vi "parser.vi"(0 "in string":string, 3 "variables":dbl[](array[numeric])=[0.0, 0.0, 0.0], 4 "leaves":string[](array[string])=["Cube", "Pyramid", "Sphere"]) -> (5 "leaves_projection_array":cluster{"matrix":dbl[][], "leave":string}[](array[cluster])=[{"matrix"=[[100.0, -1.3951473992034527e-14, -1.3951473992034527e-14, 0.0], [1.3951473992034527e-14, 100.0, -1.3951473992034527e-14, 0.0], [1.3951473992034527e-14, 1.3951473992034527e-14, 100.0, 0.0], [0.0, 0.0, 0.0, 1.0]], "leave"="Pyramid"}, {"matrix"=[[10.0, -6.975736996017264e-16, -6.975736996017264e-16, 146.93877551020412], [6.975736996017264e-16, 10.0, -6.975736996017264e-16, 10.00000000000001], [6.975736996017264e-16, 6.975736996017264e-16, 10.0, 10.00000000000001], [0.0, 0.0, 0.0, 1.0]], "leave"="Cube"}, {"matrix"=[[10.0, -6.975736996017264e-16, -6.975736996017264e-16, 9.999999999999996], [6.975736996017264e-16, 10.0, -6.975736996017264e-16, 50.0], [6.975736996017264e-16, 6.975736996017264e-16, 10.0, 10.000000000000004], [0.0, 0.0, 0.0, 1.0]], "leave"="Cube"}] {"matrix" format="%#.6f"})   [LabVIEW 2011]
uses:
  <vilib>/Analysis/baseanly.llb/Real A x B.vi
  <vilib>/Analysis/NI_AALBase.lvlib
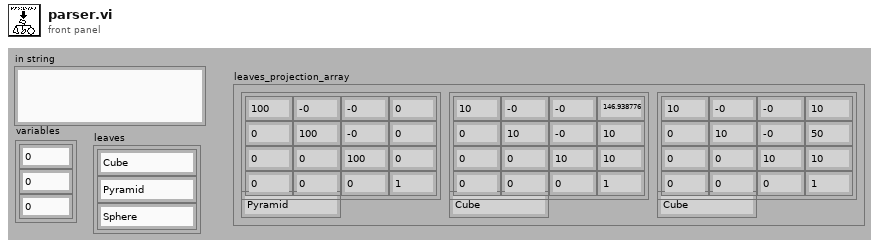
[diagram p1: front panel]
types:
  T1 = typedef "NI_Matrix.lvlib/RealMatrix.ctl" = dbl[][]
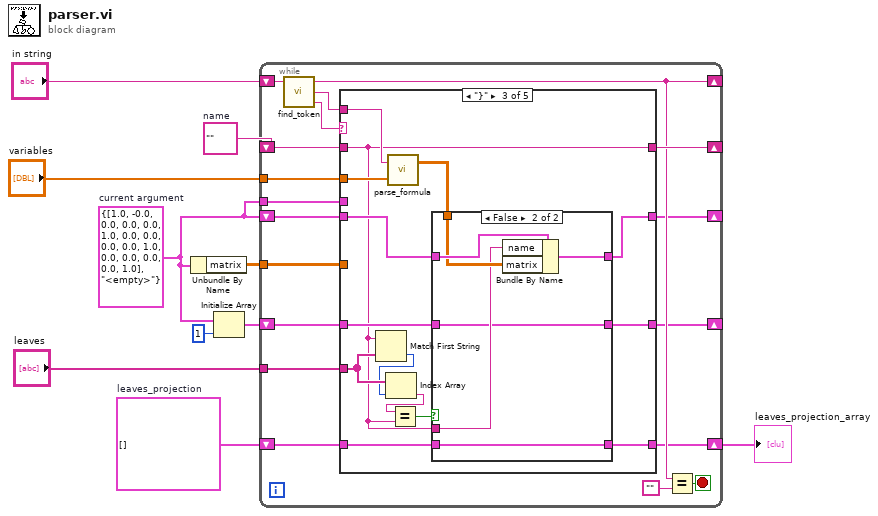
[diagram p0: block diagram]
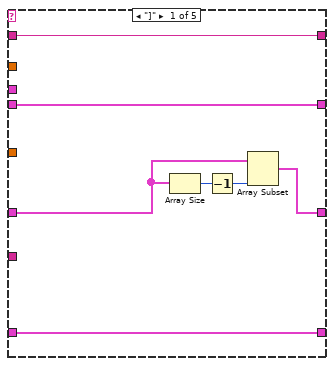
[diagram p2: hidden frame]
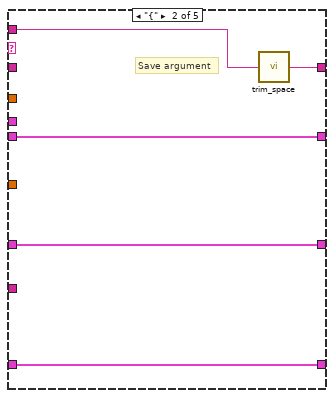
[diagram p3: hidden frame]
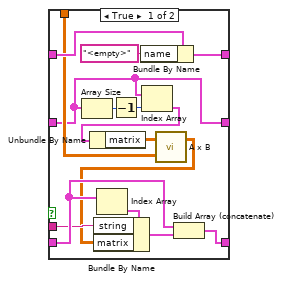
[diagram p4: hidden frame]
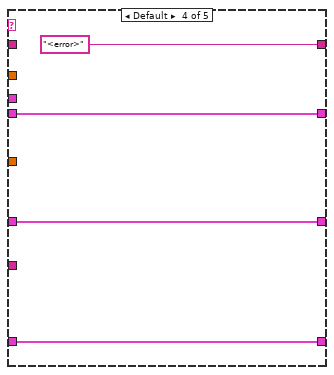
[diagram p5: hidden frame]
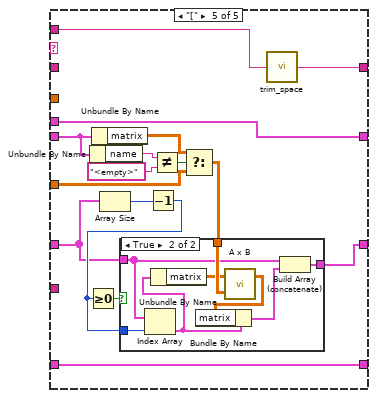
[diagram p6: hidden frame]
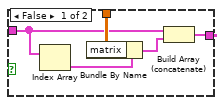
[diagram p7: hidden frame]
diagram:
  w8 = cluster{"matrix":dbl[][], "string":string}[] []  # leaves_projection
  w1 = cluster{"matrix":dbl[][], "name":string} {"matrix"=[[1.0, -0.0, 0.0, 0.0], [0.0, 1.0, 0.0, 0.0], [0.0, 0.0, 1.0, 0.0], [0.0, 0.0, 0.0, 1.0]], "name"="<empty>"}  # current argument
  w6 = ""  # name
  n1 = Unbundle By Name(w1) -> ("matrix"=w3:dbl[][])
  n2 = Initialize Array(w1, 1 ("dimension size")) -> (w7:cluster{"matrix":dbl[][], "name":string}[])
  n3 = while {
    shift-right: [w23] -> _
    shift-left: w6 -> [w24]
    shift-right: [w21] -> _
    shift-left: "in string" -> [w26]
    shift-right: [w19] -> _
    shift-left: w1 -> [w20]
    shift-right: [w17] -> _
    shift-left: w7 -> [w18]
    shift-right: [w15] -> w9
    shift-left: w8 -> [w16]
    tunnel: "leaves" -> [w14]
    tunnel: "variables" -> [w13]
    tunnel: w3 -> [w12]
    tunnel: w1 -> [w11]
    stop <- w27 stop-if-true
    n4 = call "find_token.vi"("string in"=w26) -> ("found token"=w25:string, "string before token"=w22:string, "string after token"=w21:string)  [unwired: 2 in]
    n5 = case shown="\"}\"" w25 {
      tunnel: w24 -> [w35 _ w42 _ _]
      tunnel: [w35 w36 w42 "<error>" ("string before token") w81] -> w23
      tunnel: w22 -> [_ w37 w50 _ w82]
      tunnel: w20 -> [w34 w40 w52 w78 w87]
      tunnel: [w34 w40 w51 w78 w80] -> w19
      tunnel: w18 -> [w30 w39 w47 w77 w92]
      tunnel: [w31 w39 w46 w77 w91] -> w17
      tunnel: w16 -> [w29 w38 w54 w76 w90]
      tunnel: [w29 w38 w53 w76 w90] -> w15
      tunnel: w14 -> [_ _ w45 _ _]
      tunnel: w13 -> [_ _ w48 _ _]
      tunnel: w12 -> [_ _ _ _ w85]
      tunnel: w11 -> [_ _ _ _ w80]
      frame "]" {
        n6 = Array Size(array=w30) -> (size(s)=w33:i32)
        n7 = Decrement(x=w33) -> (x-1=w32:i32)
        n8 = Array Subset(array=w30, length=w32) -> (w31:cluster{"matrix":dbl[][], "name":string}[])  [unwired: 1 in]
      }
      frame "{" {
        # "Save argument"
        n9 = call "trim_space.vi"("string in"=w37) -> ("string out"=w36:string)
      }
      frame "}" {
        n10 = Match First String(2:w45, 3:w42) -> (0:w44:i32)  [unwired: 1 out]
        n11 = Index Array(array=w45, index=w44) -> (element=w43:string)
        n12 = call "parse_formula.vi"("Vi"=w48, "formula"=w50) -> ("result matrix"=w49:dbl[][])  [unwired: 1 in]
        n13 = Equal?(x=w43, y=w42) -> (x = y?=w41:bool)
        n14 = case shown="False" w41 {
          tunnel: w54 -> [w64 w75]
          tunnel: [w65 w75] -> w53
          tunnel: w52 -> [w63 w73]
          tunnel: [w62 w74] -> w51
          tunnel: w49 -> [w60 w72]
          tunnel: w42 -> [w59 w71]
          tunnel: w47 -> [w55 w70]
          tunnel: [w55 w70] -> w46
          frame True {
            n15 = Array Size(array=w55) -> (size(s)=w67:i32)
            n16 = Index Array(array=w64) -> (element=w68:cluster{"matrix":dbl[][], "string":string})  [unwired: 1 in]
            n17 = Decrement(x=w67) -> (x-1=w66:i32)
            n18 = Bundle By Name(cluster=w63, "name"="<empty>") -> (w62:cluster{"matrix":dbl[][], "name":string})
            n19 = Index Array(array=w55, index=w66) -> (element=w56:cluster{"matrix":dbl[][], "name":string})
            n20 = Unbundle By Name(w56) -> ("matrix"=w58:dbl[][])
            n21 = call-poly <vilib>:"A x B.vi"("B"=w60, "A"=w58) -> ("A x B"=w57:T1)  [unwired: 1 out]
            n22 = Bundle By Name(cluster=w68, "string"=w59, "matrix"=w57) -> (w69:cluster{"matrix":dbl[][], "string":string})
            n23 = Build Array (concatenate)(w64, w69) -> (w65:cluster{"matrix":dbl[][], "string":string}[])
          }
          frame False {
            n24 = Bundle By Name(cluster=w73, "name"=w71, "matrix"=w72) -> (w74:cluster{"matrix":dbl[][], "name":string})
          }
        }
      }
      frame Default {
      }
      frame "[" {
        n25 = Unbundle By Name(w87) -> ("name"=w89:string)
        n26 = Unbundle By Name(w87) -> ("matrix"=w86:dbl[][])
        n27 = Array Size(array=w92) -> (size(s)=w95:i32)
        n28 = Decrement(x=w95) -> (x-1=w93:i32)
        n29 = Greater Or Equal To 0?(x=w93) -> (x >= 0?=w94:bool)
        n30 = Not Equal?(x=w89, y="<empty>") -> (x != y?=w83:bool)
        n31 = Select(t=w86, s=w83, f=w85) -> (s? t:f=w84:dbl[][])
        n32 = case shown="True" w94 {
          tunnel: [w99 w104] -> w91
          tunnel: w84 -> [w98 w108]
          tunnel: w92 -> [w96 w105]
          tunnel: w93 -> [_ w103]
          frame False {
            n33 = Index Array(array=w96) -> (element=w97:cluster{"matrix":dbl[][], "name":string})  [unwired: 1 in]
            n34 = Bundle By Name(cluster=w97, "matrix"=w98) -> (w100:cluster{"matrix":dbl[][], "name":string})
            n35 = Build Array (concatenate)(w96, w100) -> (w99:cluster{"matrix":dbl[][], "name":string}[])
          }
          frame True {
            n36 = Index Array(array=w105, index=w103) -> (element=w106:cluster{"matrix":dbl[][], "name":string})
            n37 = Unbundle By Name(w106) -> ("matrix"=w107:dbl[][])
            n38 = call-poly <vilib>:"A x B.vi"("B"=w108, "A"=w107) -> ("A x B"=w101:T1)  [unwired: 1 out]
            n39 = Bundle By Name(cluster=w106, "matrix"=w101) -> (w102:cluster{"matrix":dbl[][], "name":string})
            n40 = Build Array (concatenate)(w105, w102) -> (w104:cluster{"matrix":dbl[][], "name":string}[])
          }
        }
        n41 = call "trim_space.vi"("string in"=w82) -> ("string out"=w81:string)
      }
    }
    n42 = Equal?(x=w21, y="") -> (x = y?=w27:bool)
  }
  "leaves_projection_array" <- w9
